vi "create_document.vi"(0 "text":string, 5 "metadatas":cluster{"key":string, "value":string}[](array[cluster]), 11 "error in (no error)":errorcluster) -> (4 "data_document out":refnum<class "data_document.lvclass">, 15 "error out":errorcluster)   [LabVIEW 2020, in "data_document.lvclass"]
uses:
  data_document.lvclass
  data_document.lvclass/data_document.ctl
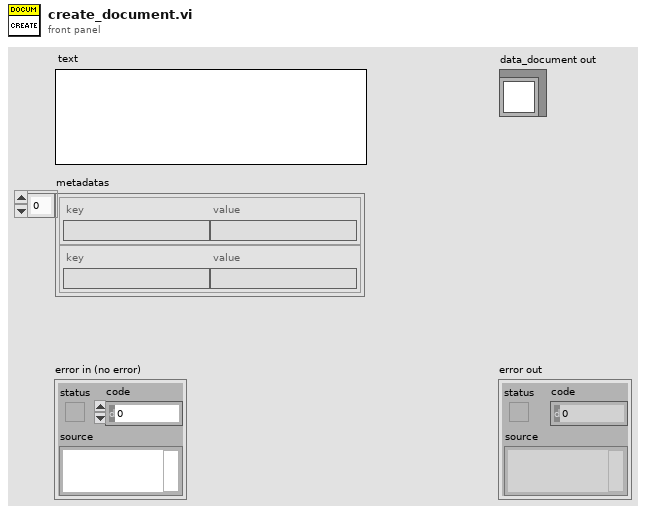
[diagram p1: front panel]
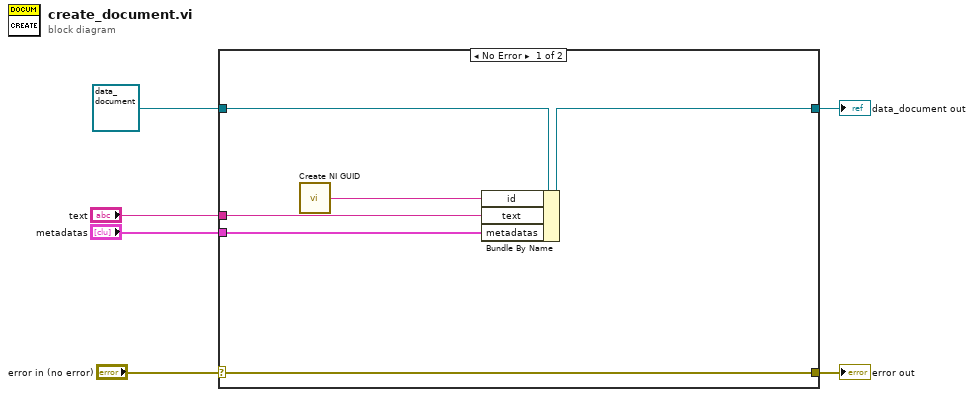
[diagram p0: block diagram]
diagram:
  n1 = case shown="No Error" "error in (no error)" {
    selector: "error in (no error)" -> [w12 w14]
    tunnel: [w12 w14] -> w5
    tunnel: [w9 w13] -> w3
    tunnel: refnum<class "data_document.lvclass"> refnum ("data_document in") -> [w11 w13]
    tunnel: "text" -> [w8 _]
    tunnel: "metadatas" -> [w7 _]
    frame No Error {
      n2 = call <vilib>:"Create NI GUID.vi"() -> ("NI GUID"=w10:string)
      n3 = Bundle By Name(cluster=w11, "id"=w10, "text"=w8, "metadatas"=w7) -> (w9:refnum<class "data_document.lvclass">)
    }
    frame Error {
    }
  }
  "error out" <- w5
  "data_document out" <- w3
